vi "GEvt-Generate with Rule Check.vi"(7 "LogFilter in":refnum<class "LogFilter.lvclass">, 10 "event data":T1, 11 "CSM Global Log Event in":refnum<user-event>) -> (3 "CSM Global Log Event out":refnum<user-event>)   [LabVIEW 2020, in "Communicable State Machine.lvlib"]
uses:
  Communicable State Machine.lvlib
  _CSM_GlobalLog_MSG.ctl
  _CSM_Response Source Message.ctl
  _CSM_GlobalLog_MSG_TYPE.ctl
  LogFilter.lvclass
  Group Check - CSM.vi
  Group Check - LogType.vi
  Group Check - State.vi
  CSM Check - LogType.vi
  CSM Check - State.vi
  CSM Check - StateType.vi
  Group Check - StateType.vi
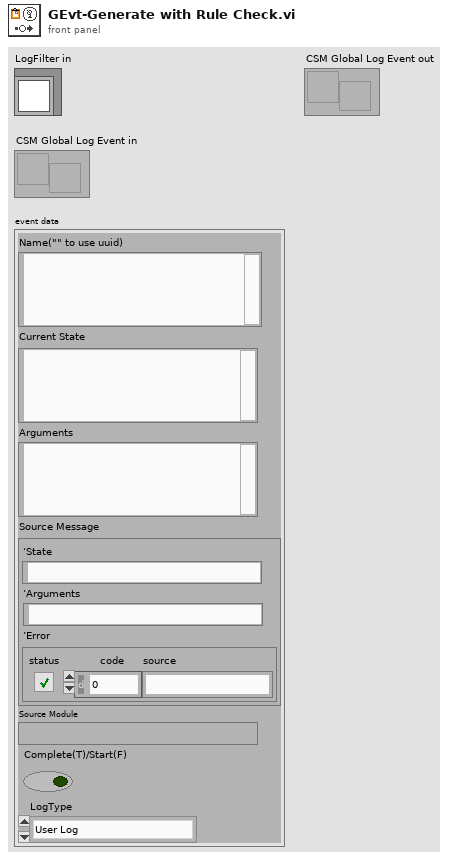
[diagram p1: front panel]
types:
  T1 = typedef "Communicable State Machine.lvlib/_CSM_GlobalLog_MSG.ctl" = cluster{"Name(\"\" to use uuid)":string, "Current State":string, "Arguments":string, "Source Message":T2, "Source Module":string, "Complete(T)/Start(F)":bool, "LogType":T3}
  T2 = typedef "Communicable State Machine.lvlib/_CSM_Response Source Message.ctl" = cluster{"‘State":string, "’Arguments":string, "’Error":errorcluster}
  T3 = typedef "Communicable State Machine.lvlib/_CSM_GlobalLog_MSG_TYPE.ctl" = enum16{"User Log", "State Change", "Status", "Interrupt", "Register", "Unregister", "Error Log", "Module Created", "Module Destroyed"}
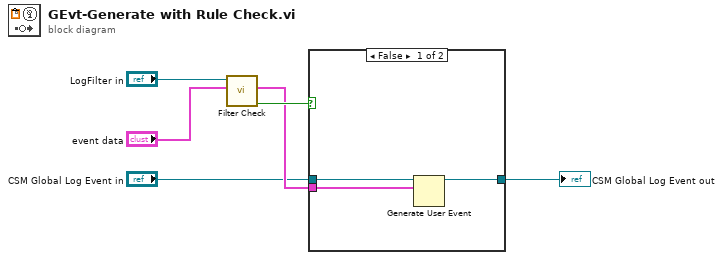
[diagram p0: block diagram]
diagram:
  n1 = call "Filter Check.vi"("Cross CSM Data in"="event data", "GlobalLogFilter in"="LogFilter in") -> ("Matched? (dup)"=w6:bool, "Cross CSM Data out"=w5:T1)  [unwired: 7 in, 1 out]
  n2 = case shown="False" w6 {
    tunnel: "CSM Global Log Event in" -> [w9 w10]
    tunnel: [w8 w10] -> w2
    tunnel: w5 -> [w7 _]
    frame False {
      n3 = Generate User Event(user event=w9, event data cluster=w7) -> (user event out=w8:refnum<user-event>)  [unwired: 2 in, 1 out]
    }
    frame True {
    }
  }
  "CSM Global Log Event out" <- w2
